vi "MathScriptODE_Test.vi"() -> ()   [LabVIEW 2014]
uses:
  <vilib>/imath/engines/lvmath/Plug In/_Char/NIMS_CH_character datatype.ctl
  <vilib>/imath/engines/lvmath2/RunTimeEngine/Managers/WorkSpace/UID Generator.vi
  <vilib>/imath/engines/lvmath/Plug In/_Char/NIMS_CH_Character RV to String.vi
  C:/Users/Wilcken/Documents/LabVIEW Data/MathScriptVIs/MCStatic_33557714032_8fc4b031efb2b45cd4d9644c72878fd3.vi
  <vilib>/imath/engines/lvmath2/RunTimeEngine/BuiltInFunctions/ode_adams/NIMS_[RV,RM]=ode_adams.vi
  <vilib>/imathl/engines/lvmath/Functions/Error Handling/Create Error.vi
  <vilib>/imath/engines/lvmath2/RunTimeEngine/Managers/SymbolTable/Clear UID.vi
  <vilib>/imath/engines/lvmath2/RunTimeEngine/NodeEndStatement/NIMS_NodeEndStatement_Output.vi
  <instcachedir>/0/NIMS_NodeEndStatement_Output_53EC0D466D134D7ABD903AC30B43404B.lvgen/NIMS_NodeEndStatement_Output_53EC0D466D134D7ABD903AC30B43404B_002.vi
  <instcachedir>/0/NIMS_NodeEndStatement_Output_53EC0D466D134D7ABD903AC30B43404B.lvgen/NIMS_NodeEndStatement_Output_53EC0D466D134D7ABD903AC30B43404B_005.vi
  <vilib>/imath/engines/lvmath2/RunTimeEngine/ErrorHandling/NIMS_Finalize Error.vi
  C:/Users/Wilcken/Desktop/model.m
  <vilib>/imath/engines/lvmath2/RunTimeEngine/Managers/SymbolTable/NIMS_WorkSpace.lvlib
panel:
  out "XY Graph":cluster{"Times":dbl[], "X Values":dbl[]}[](graph)
  out "N":dbl[][](array[numeric])
  out "t 3":dbl[](array[numeric])
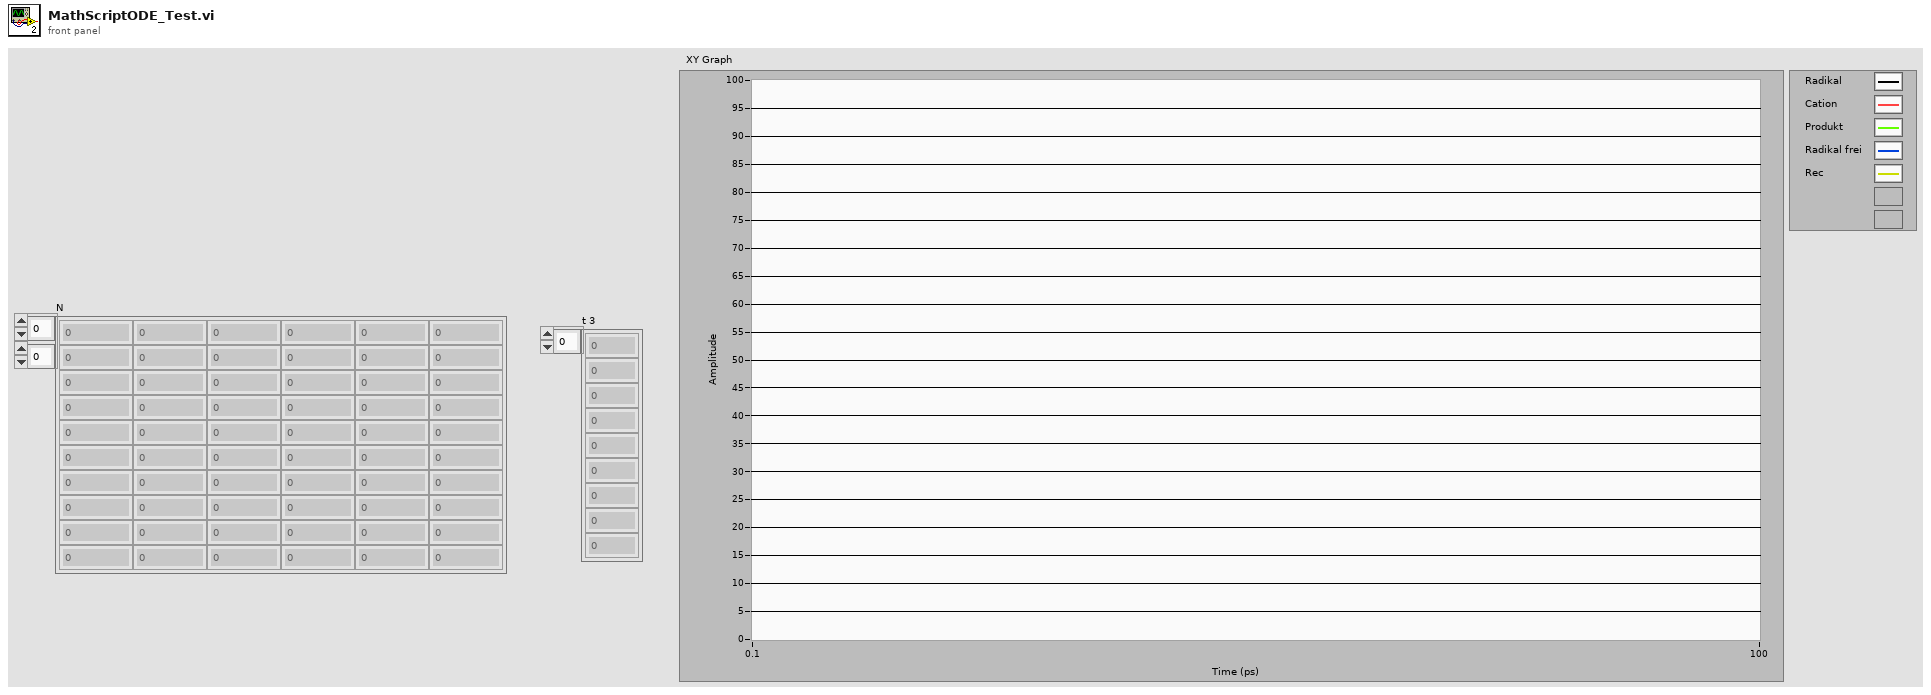
[diagram p1: front panel]
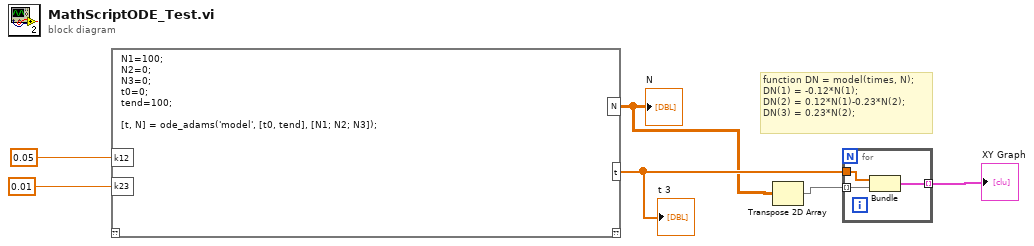
[diagram p0: block diagram]
diagram:
  # "function DN = model(times, N);\nDN(1) = -0.12*N(1);\nDN(2) = 0.12*N(1)-0.23*N(2);\nDN(3) = 0.23*N(2);"
  n1 = mathscript code="N1=100;\nN2=0;\nN3=0;\nt0=0;\ntend=100;\n\n[t, N] = ode_adams('model', [t0, tend], [N1; N2; N3]);"("k12"=0.05, "k23"=0.01) -> ("t"=w6:dbl[], "N"=w4:dbl[][])  [unwired: 1 in, 1 out]
  "t 3" <- w6
  "N" <- w4
  n2 = Transpose 2D Array(2D array=w4) -> (transposed array=w3:dbl[][])
  n3 = for {
    tunnel: w3 -> [w9] mode=indexing
    tunnel: w6 -> [w8]
    tunnel: [w7] -> w5 mode=indexing
    n4 = Bundle("t"=w8, w9) -> (w7:cluster{"t":dbl[], dbl[]})  [unwired: 1 in]
  }
  "XY Graph" <- w5
